vi "Exemple_Metrics_Contingency_Matrix.vi"() -> ()   [LabVIEW 2020]
uses:
  Objet/3 - Model selection and evaluation/3.3 - Metrics and scoring/contingency_matrix/Contingency_Matrix.vi
panel:
  out "Data":T1
  out "error out":errorcluster caption="sortie d'erreur"
  in  "error in (no error)":errorcluster caption="entrée d'erreur (pas d'erreur)"
  in  "contingency_matrix":cluster{"eps":string, "sparse":bool}={"eps"="None", "sparse"=FALSE}
  in  "labels_pred":string[][](array[string])=[["0"], ["0"], ["1"], ["1"], ["2"], ["2"]]
  in  "labels_true":string[][](array[string])=[["a"], ["a"], ["a"], ["b"], ["b"], ["b"]]
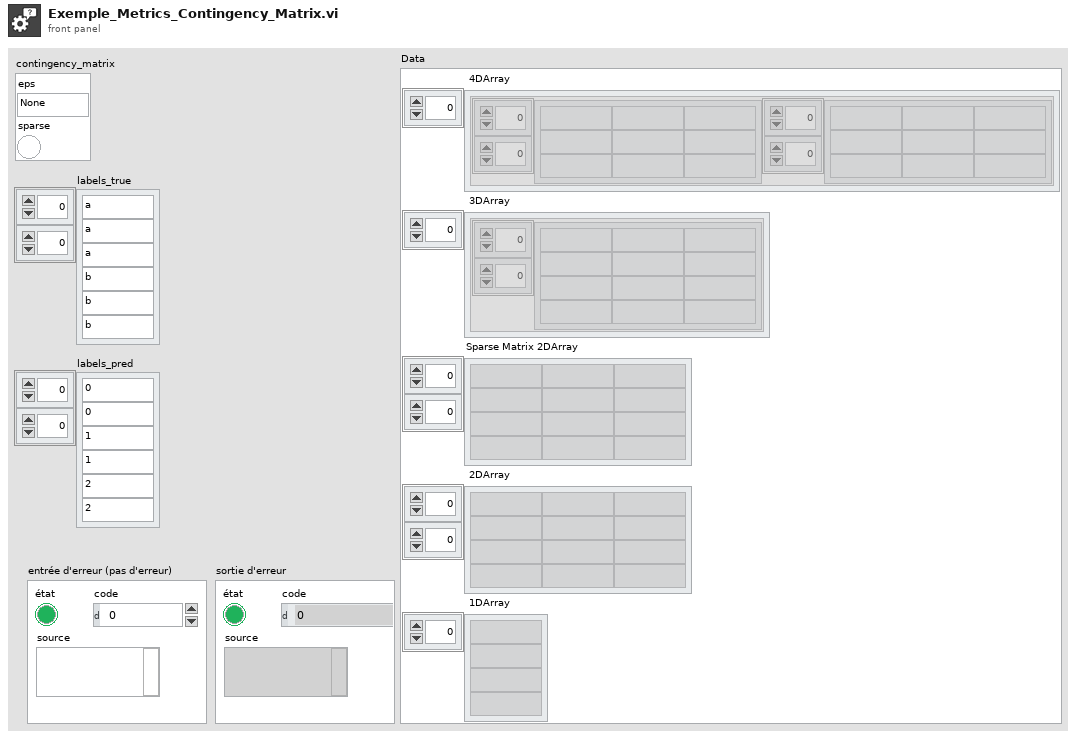
[diagram p1: front panel]
types:
  T1 = cluster{" 4DArray":cluster{"1":string[][], "2":string[][]}[], " 3DArray":cluster{"Tableau":string[][]}[], "Sparse Matrix 2DArray":string[][], " 2DArray":string[][], " 1DArray":string[]}
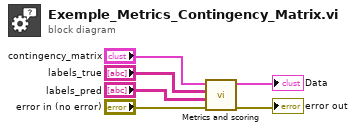
[diagram p0: block diagram]
diagram:
  n1 = call-poly "Metrics and scoring.vi"("error in (no error)"="error in (no error)", "labels_pred"="labels_pred", "labels_true"="labels_true", "contingency_matrix"="contingency_matrix") -> ("error out"=→"error out":errorcluster, "Data"=→"Data":T1)  [unwired: 6 in]
